vi "MAIN - Quick VIew.vi"() -> ()   [LabVIEW 2014, in "QuickVIew.lvlib"]
uses:
  QuickVIew.lvlib
  Components/System Triggers.ctl
  Components/State Declaration.ctl
  Components/Tree Control/Typedef/TYPEDEF - DataStore Command.ctl
  <vilib>/Utility/error.llb/DialogTypeEnum.ctl
  <vilib>/NI/AMC/Read Termination Message.vi
  <vilib>/NI/AMC/Update Message Routing Info.vi
  <vilib>/NI/AMC/Create Multiple Messages.vi
  <vilib>/NI/AMC/Create Single Message.vi
  Components/TypeDef - SHIFTER.ctl
  <vilib>/NI/AMC/Globals.vi
  Components/VI Collection/set Active VIs.vi
  <vilib>/NI/AMC/Send Message.vi
  <vilib>/LabVIEW Icon API/lv_icon/Classes/Icon/Icon.lvclass
  Components/VI Collection/VI Collection.lvclass
  Components/Dependencies.llb/TLB`_Dependencies.lvlib
  <vilib>/NI/AMC/AMC.lvlib
  <vilib>/LabVIEW Icon API/LabVIEW Icon API.lvlib
panel:
  out "Active Icon":picture
  in  "Settings Button":bool
  in  "Unload Button":bool
  in  "Load Button":bool
  in  "Collection View":string(tree)
  in  "DEBUG::VIew Item":enum16{"Block Diagram", "Front Panel", "Icon"}(ring)
  in  "Send Trigger":bool
  in  "System Triggers":T1=enum."Load Selection"
  out "error out":errorcluster
  # "Quick VIew"
  # "Debug Pane"
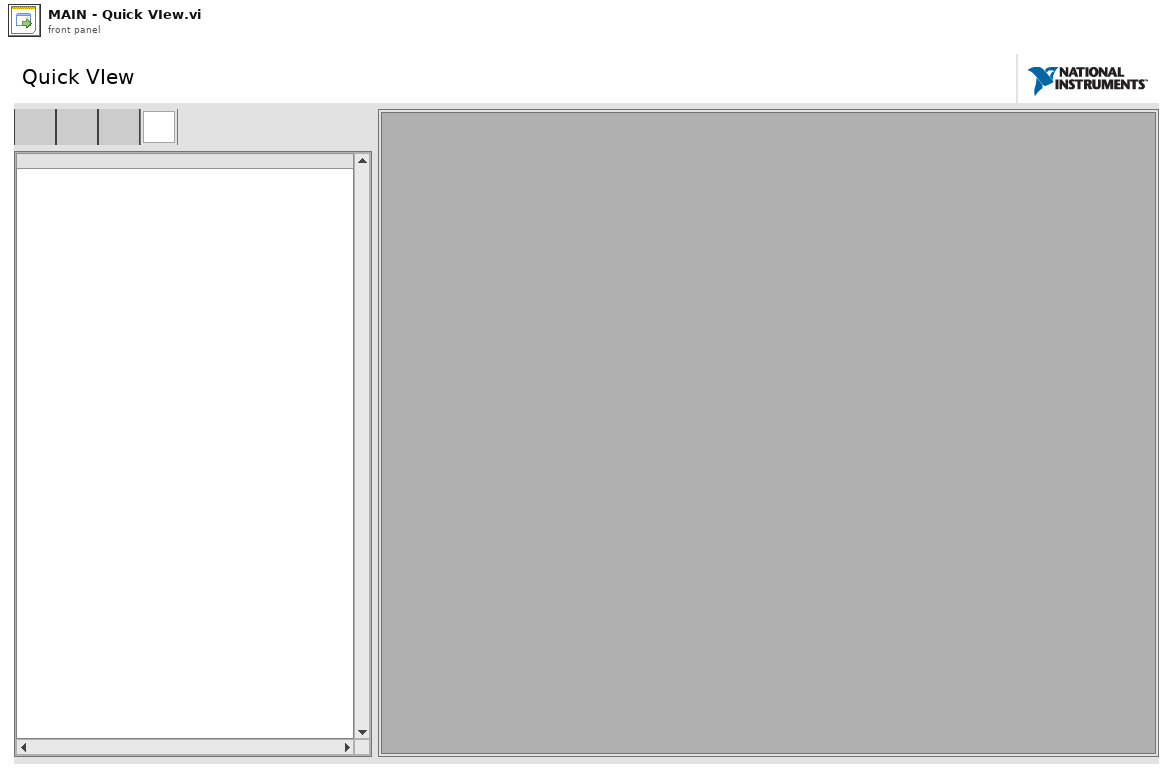
[diagram p1: front panel]
types:
  T1 = typedef "QuickVIew.lvlib/System Triggers.ctl" = enum16{"<None>", "Cache User Parameters", "Close Application", "---------------------------", "Change VI", "Open Current VI", "Save VI", "Unload Collection", "Load Selection", "Edit Icon"}
  T2 = enum16{"Clear SR", "Set Display", "Set Shifter", "Initialize Events", "Init Q"}
  T3 = typedef "QuickVIew.lvlib/TypeDef - SHIFTER.ctl" = cluster{"State":T4, "User Data":cluster{"Active Item Tag":string}, "Display Data":cluster{"Current Project Name":string, "Active Icon":picture}, "User Parameter Controls":refnum<vi>[], "Framework Data":cluster{"Exit Event":T5, "Terminate Error":errorcluster}, "Private Data":cluster{"Active Item Tag":string, "Scroll Event":refnum<user-event>, "ActiveProject":refnum<vi>, "Active VI":cluster{"App Ref":refnum<vi>, "VI Name":string, "Active Window":enum16{"FP", "BD"}, "Icon":refnum<class "Icon.lvclass">}, "Loaded VI":refnum<vi>, "Collection View Tree":refnum<vi>, "Item View":refnum<vi>, "VI Collection":refnum<class "VI Collection.lvclass">}}
  T4 = typedef "QuickVIew.lvlib/State Declaration.ctl" = enum16{"<Startup>", "Idle", "<Shutdown>", "-", "Viewing"}
  T5 = typedef "QuickVIew.lvlib/TLB`_Dependencies.lvlib/Exit Event Ref.ctl" = refnum<user-event>
  T6 = typedef "AMC.lvlib/Message Queue.ctl" = refnum<queue>
  T7 = typedef "QuickVIew.lvlib/TYPEDEF - DataStore Command.ctl" = enum16{"Init", "Add", "Get", "Clear Tree", "Clear All", "Modify"}
  T8 = enum32{"Invalid", "Standard", "Closed", "Hidden", "Minimized", "Maximized"}
  T9 = typedef "DialogTypeEnum.ctl" = enum16{"no dialog", "OK message", "continue or stop message", "auto error handling dialog", "OK message + warnings", "continue/stop + warnings"}
  T10 = typedef "imagedata.ctl" = cluster{"image type":i32, "image depth":i32, "image":u8[], "mask":u8[], "colors":u32[], "Rectangle":cluster{"left":i16, "top":i16, "right":i16, "bottom":i16}}
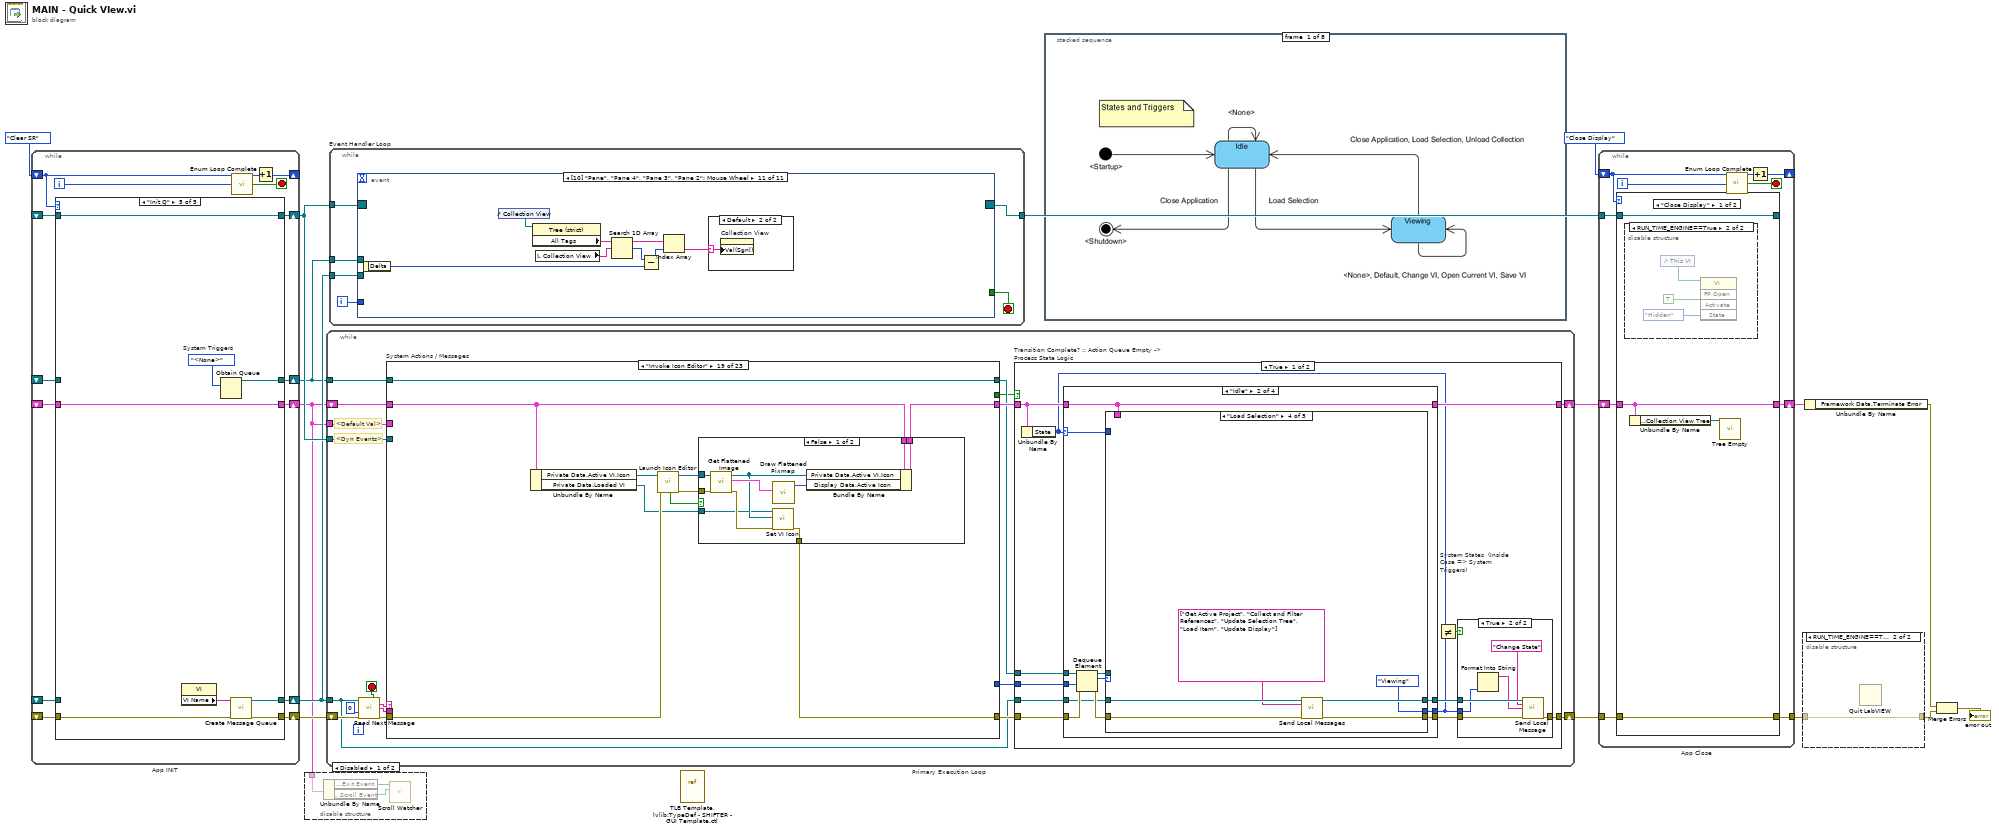
[diagram p0: block diagram]
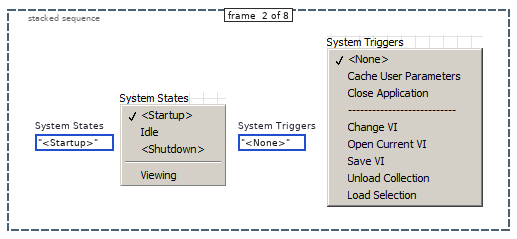
[diagram p3: hidden frame]
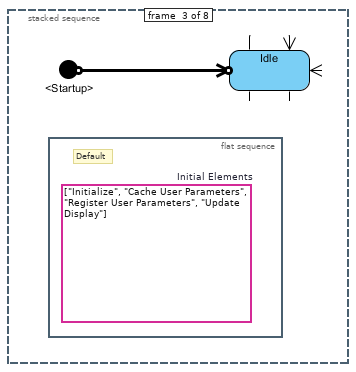
[diagram p4: hidden frame]
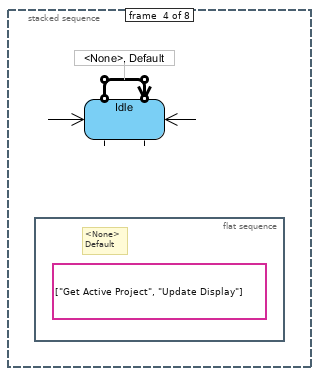
[diagram p5: hidden frame]
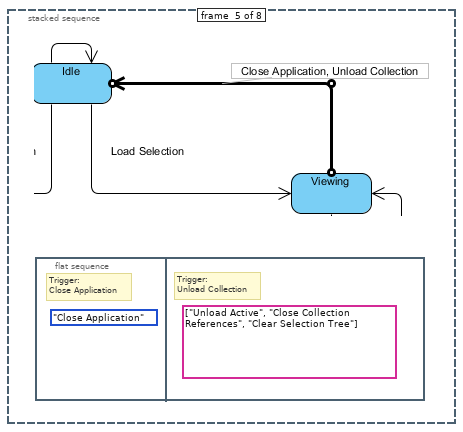
[diagram p6: hidden frame]
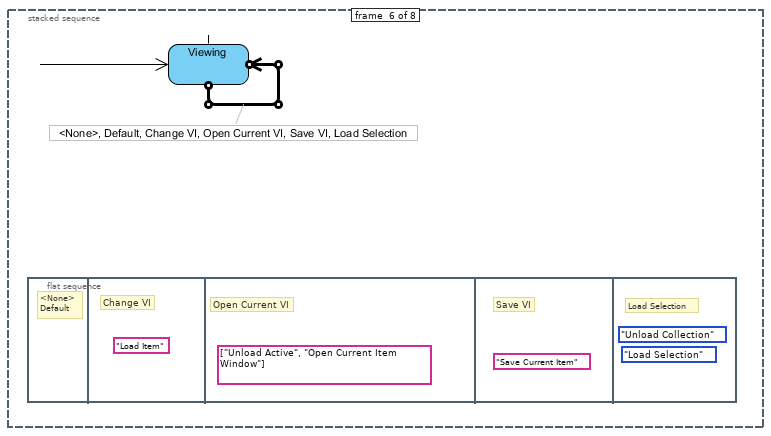
[diagram p7: hidden frame]
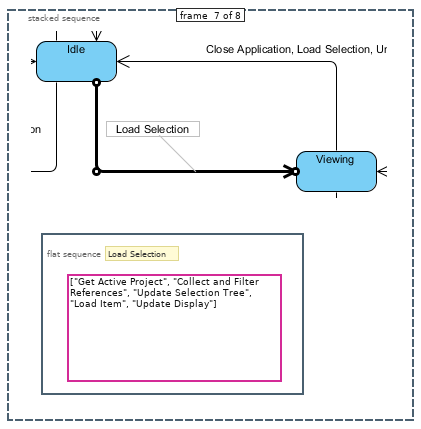
[diagram p8: hidden frame]
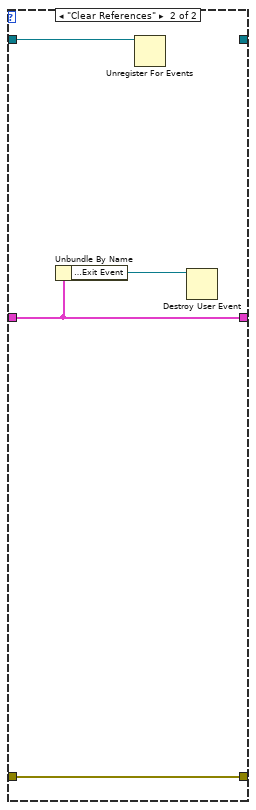
[diagram p12: hidden frame]
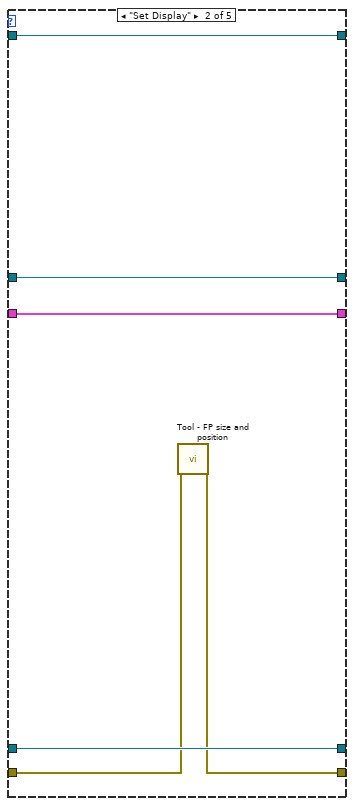
[diagram p14: hidden frame]
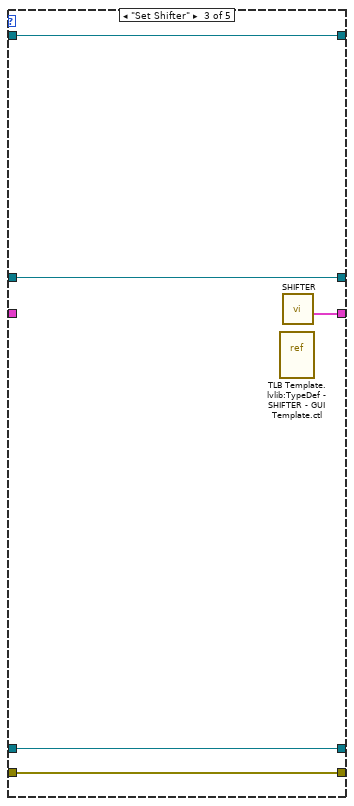
[diagram p15: hidden frame]
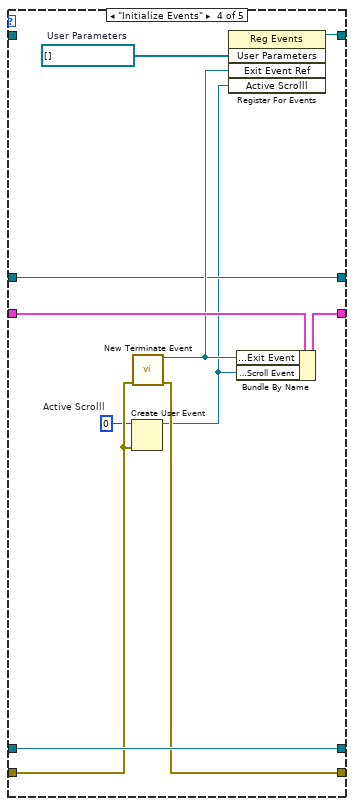
[diagram p16: hidden frame]
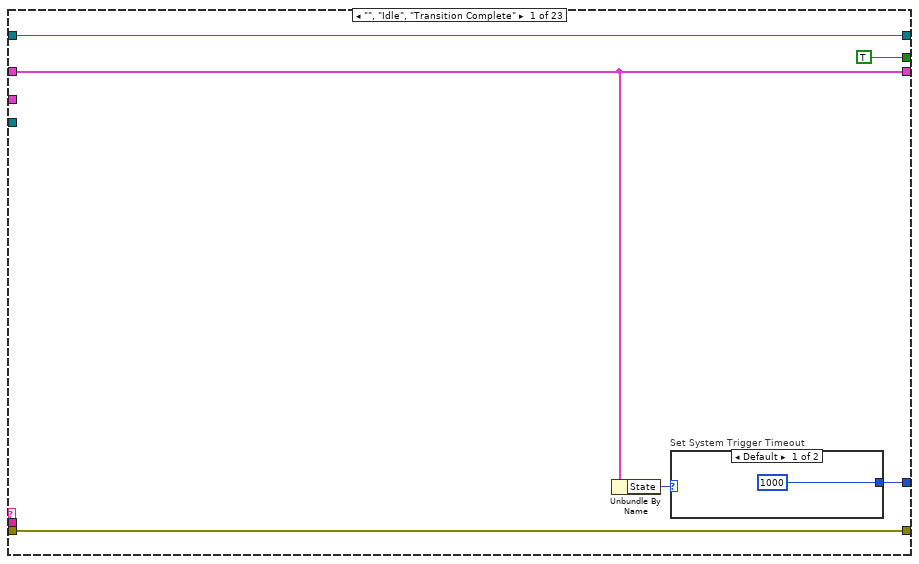
[diagram p17: hidden frame]
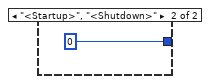
[diagram p18: hidden frame]
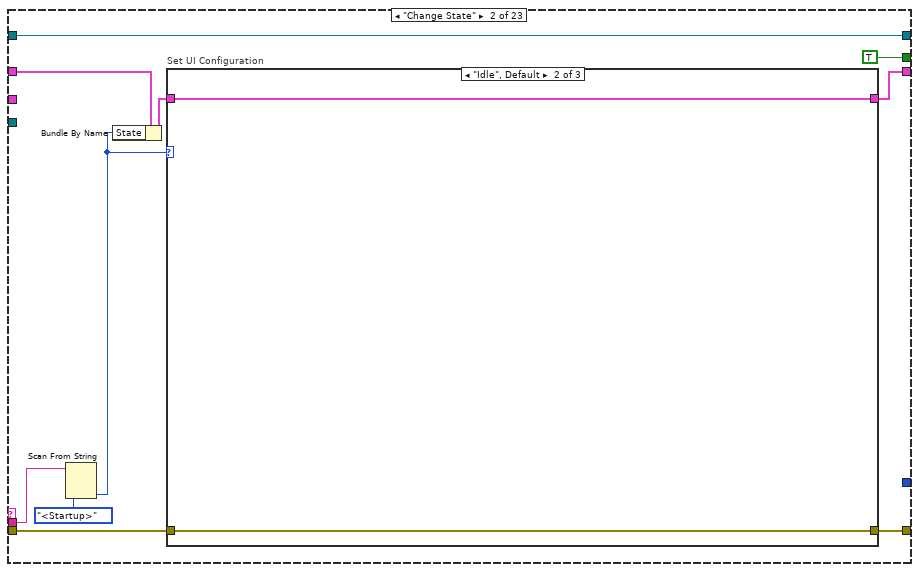
[diagram p19: hidden frame]
diagram:
  n1 = while "App INIT" {
    shift-right: [w23] -> _
    shift-left: T2."Clear SR" -> [w18]
    shift-right: [w29] -> w9
    shift-left: _ -> [w22]
    shift-right: [w26] -> w8
    shift-left: _ -> [w21]
    shift-right: [w28] -> w11
    shift-left: _ -> [w20]
    shift-right: [w27] -> w1
    shift-left: _ -> [w19]
    shift-right: [w17] -> w2
    shift-left: _ -> [w16]
    i -> [w24]
    stop <- w25 stop-if-true
    n2 = case shown="\"Init Q\"" w18 {
      tunnel: [_ w33 w40 w51 w56] -> w29
      tunnel: [_ w31 w39 w45 w54] -> w26
      tunnel: [_ w35 w36 w48 w58] -> w27
      tunnel: [_ w34 w38 w47 w59] -> w28
      tunnel: w22 -> [_ w33 w40 w51 _]
      tunnel: w21 -> [_ w32 w39 w43 w55]
      tunnel: w20 -> [_ w34 w38 _ w59]
      tunnel: w19 -> [_ w35 _ w49 w58]
      tunnel: [_ w30 w37 w44 w53] -> w17
      tunnel: w16 -> [_ w30 w37 w44 _]
      frame "Clear SR" {
      }
      frame "Set Display" {
        n3 = call "Tool - FP size and position.vi"("error in (no error)"=w32) -> ("error out"=w31:errorcluster)  [unwired: 7 in, 11 out]
      }
      frame "Set Shifter" {
        n4 = vi-ref "TLB Template.lvlib:TypeDef - SHIFTER - GUI Template.ctl"() -> ()  [unwired: 1 out]
        n5 = call "SHIFTER.vi"() -> ("SHIFTER DATA"=w36:T3)  [unwired: 15 in]
      }
      frame "Initialize Events" {
        w41 = i16 0  # Active Scrolll
        w50 = refnum<vi>[] []  # User Parameters
        n6 = Create User Event(user event datatype=w41, error in=w43) -> (user event=w42:refnum<user-event>)  [unwired: 1 out]
        n7 = call "New Terminate Event.vi"("error in (no error)"=w43) -> ("Exit Event Ref"=w46:T5, "error out"=w45:errorcluster)  [unwired: 13 in]
        n8 = register-events(w50, w46, w42) -> (reference out=w47:refnum<event-registration>)  [unwired: 2 in, 1 out]
        n9 = Bundle By Name(cluster=w49, "Framework Data.Exit Event"=w46, "Private Data.Scroll Event"=w42) -> (w48:T3)
      }
      frame "Init Q" {
        w52 = System_Triggers."<None>"  # System Triggers
        n10 = property class="VI"() -> ("VI Name"=w57:string)  [unwired: 2 in, 2 out]
        n11 = Obtain Queue(element data type=w52) -> (queue out=w53:refnum<queue>)  [unwired: 4 in, 2 out]
        n12 = call <vilib>:"Create Message Queue.vi"("message queue name"=w57, "error in"=w55) -> ("message queue out"=w56:T6, "error out"=w54:errorcluster)  [unwired: 12 in]
      }
    }
    n13 = call "Enum Loop Complete.vi"("Current State Enum"=w18, "Itteration"=w24) -> ("Loop Complete?"=w25:bool)  [unwired: 13 out]
    n14 = Increment(x=w18) -> (x+1=w23:T2)
  }
  n15 = disable-structure shown="Disabled" {
    disable-tunnel: w1 -> [w62 _]
    frame Disabled {
      n16 = Unbundle By Name(w62) -> ("Framework Data.Exit Event"=w61:T5, "Private Data.Scroll Event"=w60:refnum<user-event>)
      n17 = call "Scroll Watcher.vi"("Exit Command"=w61, "NewVal"=w60) -> ()  [unwired: 14 in]
    }
    frame Enabled {
    }
  }
  n18 = while "Primary Execution Loop" {
    shift-right: [w70] -> w15
    shift-left: w8 -> [w77]
    shift-right: [w73] -> w14
    shift-left: w1 -> [w80]
    tunnel: w1 -> [w79]
    tunnel: w9 -> [w68]
    tunnel: w11 -> [w78]
    tunnel: w2 -> [w69]
    stop <- w75 stop-if-true
    # "<Dyn Events>"
    # "<Default Val>"
    n19 = call <vilib>:"Read Next Message.vi"("message queue in"=w68, "timeout (1 ms)"=0 ("timeout (1ms)"), "error in"=w77) -> ("exit process?"=w75:bool, "message name"=w74:string, "message value"=w65:string, "error out"=w76:errorcluster)  [unwired: 5 in, 4 out]
    n20 = case "System Actions / Messages" shown="\"Invoke Icon Editor\"" w74 {
      selector: w74 -> [_ _ _ _ _ _ _ _ _ _ _ _ _ _ _ _ _ _ _ _ _ _ w345]
      tunnel: [w86 w93 w107 w113 w122 w125 w130 w134 w137 w140 w189 w200 w219 w249 w261 w278 w281 w282 w290 w311 w316 w339 w349] -> w71
      tunnel: w76 -> [w86 w92 w107 w114 w122 w125 w130 w134 w137 w141 w190 w201 w220 w250 w262 w278 w281 w283 w295 w311 w317 w338 w350]
      tunnel: w80 -> [w81 w89 w106 w111 w121 w124 w128 w132 w136 w139 w194 w205 w229 w251 w263 w275 w280 w284 w294 w310 w314 w342 w351]
      tunnel: w79 -> [_ _ _ _ _ _ _ _ _ _ _ _ _ _ _ _ _ _ _ _ _ _ _]
      tunnel: [w81 w91 w106 w110 w120 w124 w127 w132 w136 w142 w193 w204 w228 w251 w263 w275 w280 w284 w293 w310 w315 w342 w351] -> w72
      tunnel: [w82 _ _ _ _ _ _ _ _ _ _ _ _ _ _ _ _ _ _ _ _ _ _] -> w64
      tunnel: w78 -> [_ _ _ _ w119 _ _ _ _ _ _ _ _ _ _ _ _ _ _ _ _ _ _]
      tunnel: [w84 w97 w105 w115 w118 w123 w129 w133 w135 w150 w197 w210 w241 w260 w274 w277 w279 w286 w296 w309 w312 w336 w343] -> w67
      tunnel: w69 -> [w84 w97 w105 w115 w118 w123 w129 w133 w135 w150 w197 w210 w241 w260 w274 w277 w279 w286 w296 w309 w312 w336 w343]
      tunnel: [TRUE TRUE _ _ _ _ _ _ _ _ _ _ _ _ _ _ _ _ _ _ _ _ _] -> w66
      tunnel: w65 -> [_ w96 _ _ _ _ _ _ _ _ _ _ _ _ _ _ _ _ _ _ _ _ _]
      frame "", "Idle", "Transition Complete" {
        n21 = Unbundle By Name(w81) -> ("State"=w83:T4)
        n22 = case "Set System Trigger Timeout" shown="Default" w83 {
          tunnel: [1000 0] -> w82
          frame Default {
          }
          frame "<Startup>", "<Shutdown>" {
          }
        }
      }
      frame "Change State" {
        n23 = Scan From String(input string=w96, default 1=State_Declaration."<Startup>" ("State")) -> (output 1=w94:T4)  [unwired: 3 in, 3 out]
        n24 = Bundle By Name(cluster=w89, "State"=w94) -> (w90:T3)
        n25 = case "Set UI Configuration" shown="\"Idle\", Default" w94 {
          tunnel: [w99 w102 w104] -> w93
          tunnel: w92 -> [w99 w102 w104]
          tunnel: [w100 w101 w103] -> w91
          tunnel: w90 -> [w100 w101 w103]
          frame "<Startup>" {
          }
          frame "Idle", Default {
          }
          frame "<Shutdown>" {
          }
        }
      }
      frame "/*********Initialize********/" {
      }
      frame "Initialize" {
        n26 = control-ref of="Collection View"() -> (w112:refnum<vi>)
        n27 = control-ref of="View Panel"() -> (w108:refnum<vi>)
        n28 = call "Tree Empty.vi"("Tree Reference In"=w112, "error in (no error)"=w114) -> ("Tree Reference Out"=w109:refnum<vi>, "error out"=w113:errorcluster)  [unwired: 15 in, 1 out]
        n29 = Bundle By Name(cluster=w111, "Private Data.Item View"=w108, "Private Data.Collection View Tree"=w109) -> (w110:T3)
      }
      frame "Register User Parameters" {
        n30 = control-ref of="Collection View"() -> (w116:refnum<vi>)
        n31 = Build Array(w116) -> (w117:refnum<vi>[])
        n32 = register-events(reference=w119, w117) -> ()  [unwired: 3 in, 2 out]
        n33 = Bundle By Name(cluster=w121, "User Parameter Controls"=w117) -> (w120:T3)
      }
      frame "/*********Display Updates********/" {
      }
      frame "Cache User Parameters" {
        n34 = Bundle By Name(cluster=w128, "User Data.Active Item Tag"="Collection View") -> (w127:T3)
      }
      frame "Update Display" {
        n35 = Unbundle By Name(w132) -> ("Display Data.Active Icon"=→"Active Icon":picture)
      }
      frame "/*********Primary Execution********/" {
      }
      frame "Get Active Project" {
        n36 = Unbundle By Name(w139) -> ("Display Data.Current Project Name"=w149:string, "Private Data.ActiveProject"=w146:refnum<vi>)
        n37 = property class="App"(error in=w141) -> (error out=w143:errorcluster, "Project.ActiveProject"=w144:refnum<vi>)  [unwired: 1 in, 1 out]
        n38 = while {
          tunnel: w139 -> [w152]
          tunnel: [w151] -> w138
          stop <- w153 stop-if-true
          n39 = event shown="[1] VI Activation" {
            selector: _ -> [_ _]
            dyn-events: _ -> [_ _]
            timeout: 0 -> [_ _]
            tunnel: [TRUE TRUE] -> w153
            tunnel: w152 -> [w155 w159]
            tunnel: [w155 w158] -> w151
            event Timeout {
              n40 = event-data() -> ()  [unwired: 1 in, 1 out]
            }
            event VI Activation {
              n41 = event-data() -> ("VIName"=w160:string, "VIAppRef"=w161:refnum<vi>, "VIWindow"=w164:i32)  [unwired: 1 in]
              n42 = property class="VI"() -> ("Name"=w163:string)  [unwired: 2 in, 2 out]
              n43 = Equal?(x=w160, y=w163) -> (x = y?=w162:bool)
              n44 = case shown="False" w162 {
                tunnel: w164 -> [w166 w174]
                tunnel: w161 -> [w167 _]
                tunnel: w160 -> [w168 _]
                tunnel: w159 -> [w170 w173]
                tunnel: [w169 w173] -> w158
                frame False {
                  n45 = case shown="1" w166 {
                    tunnel: [enum16{"FP", "BD"}."FP" enum16{"FP", "BD"}."BD"] -> w165
                    frame 0, Default {
                    }
                    frame 1 {
                    }
                  }
                  n46 = Bundle By Name(cluster=w170, "Private Data.Active VI.VI Name"=w168, "Private Data.Active VI.App Ref"=w167, "Private Data.Active VI.Active Window"=w165) -> (w169:T3)
                }
                frame True {
                  n47 = case shown="1" w174 {
                    tunnel: [enum16{"FP", "BD"}."FP" enum16{"FP", "BD"}."BD"] -> _
                    frame 0, Default {
                    }
                    frame 1 {
                    }
                  }
                }
              }
            }
          }
        }
        n48 = Equal?(x=w146, y=w144) -> (x = y?=w145:bool)
        n49 = case "is active project ref unchanged?" shown="True" w145 {
          tunnel: w144 -> [w182 w188]
          tunnel: w146 -> [w178 w187]
          tunnel: [w180 w187] -> w147
          tunnel: [w181 w186] -> w140
          tunnel: w143 -> [w183 w185]
          tunnel: [w179 w184] -> w148
          tunnel: w149 -> [_ w184]
          frame False {
            n50 = property class="Project"(reference=w182, error in=w183) -> (reference out=w180:refnum<vi>, error out=w181:errorcluster, "Name"=w179:string)
            n51 = Close Reference(reference=w178, error in (no error)=w183) -> (error out=w177:errorcluster)
            n52 = call <vilib>:"Clear Errors.vi"("error in (no error)"=w177) -> ()  [unwired: 5 in, 2 out]
          }
          frame True {
            n53 = Close Reference(reference=w188, error in (no error)=w185) -> (error out=w186:errorcluster)
          }
        }
        n54 = Bundle By Name(cluster=w138, "Display Data.Current Project Name"=w148, "Private Data.ActiveProject"=w147) -> (w142:T3)
      }
      frame "Collect and Filter References" {
        n55 = Unbundle By Name(w194) -> ("Private Data.VI Collection"=w196:refnum<class "VI Collection.lvclass">, "Private Data.ActiveProject"=w192:refnum<vi>)
        n56 = call "Harvest Selected Project Vi.vi"("ActiveProject"=w192, "error in"=w190) -> ("Array"=w191:refnum<vi>[], "error out"=w198:errorcluster)  [unwired: 12 in]
        n57 = property class="VI Collection"(reference=w196, error in=w198, "Active VIs"=w191) -> (reference out=w195:refnum<class "VI Collection.lvclass">, error out=w189:errorcluster)
        n58 = Bundle By Name(cluster=w194, "Private Data.VI Collection"=w195) -> (w193:T3)
      }
      frame "Update Selection Tree" {
        n59 = Unbundle By Name(w205) -> ("Private Data.Collection View Tree"=w206:refnum<vi>, "Private Data.VI Collection"=w199:refnum<class "VI Collection.lvclass">)
        n60 = call "get Names.vi"("error in (no error)"=w201, "VI Collection in"=w199) -> ("error out"=w202:errorcluster, "VI Ref"=w208:refnum<vi>[], "VI Names"=w207:string[])  [unwired: 6 in, 1 out]
        n61 = for {
          tunnel: w206 -> [w216]
          tunnel: w207 -> [w215] mode=indexing
          tunnel: w208 -> [w214] mode=indexing
          tunnel: [w213] -> w209 mode=indexing
          shift-right: [w211] -> w200
          shift-left: w202 -> [w212]
          n62 = call "Item Add.vi"("Tree Reference In"=w216, "New Text Value"=w215, "Tree Element Data In"=w214, "error in (no error)"=w212, "Make Top Level Item"=TRUE) -> ("Created Tag"=w213:string, "error out"=w211:errorcluster)  [unwired: 12 in, 1 out]
        }
        n63 = Index Array(array=w209) -> (element=w203:string)  [unwired: 1 in]
        n64 = local write "Collection View"(w203) -> ()
        n65 = Bundle By Name(cluster=w205, "User Data.Active Item Tag"=w203) -> (w204:T3)
      }
      frame "Load Item" {
        n66 = Unbundle By Name(w229) -> ("Private Data.Collection View Tree"=w232:refnum<vi>, "User Data.Active Item Tag"=w233:string)
        n67 = Unbundle By Name(w229) -> ("Private Data.Item View"=w231:refnum<vi>)
        n68 = call "VIG - Element DB.vi"("Tree Ref In"=w232, "Element Tag"=w233, "error in (no error)"=w220, "Command"=TYPEDEF_-_DataStore_Command."Get") -> ("Tree Element Data Out"=w234:variant, "error out"=w236:errorcluster)  [unwired: 6 in, 4 out]
        n69 = Variant To Data(error in=w236, type=refnum<vi> refnum ("Reference"), Variant=w234) -> (data=w239:refnum<vi>, error out=w240:errorcluster)
        n70 = property class="VI"(reference=w239, error in=w240, "Edit Mode"=TRUE ("Edit Mode On Open")) -> (reference out=w226:refnum<vi>, error out=w223:errorcluster)
        n71 = case shown="\"Block Diagram\", Default" "DEBUG::VIew Item" {
          tunnel: w231 -> [w245 w248]
          tunnel: w223 -> [w244 _]
          tunnel: w226 -> [w242 w247]
          tunnel: [w242 w247] -> w227
          frame "Block Diagram", Default {
            w246 = TRUE ("ShowHScrollBar")
            n72 = invoke on="Invoke Node" class="SubPanel" method="InsertBD"(reference=w245, error in=w244, "VIRef"=w242, "ShowHScrollBar?"=w246, "ShowVScrollBar?"=w246) -> (error out=w243:errorcluster)  [unwired: 1 in, 5 out]
            n73 = call <vilib>:"Clear Errors.vi"("error in (no error)"=w243) -> ()  [unwired: 5 in, 2 out]
          }
          frame "Front Panel" {
            n74 = invoke on="Invoke Node" class="SubPanel" method="Insert VI"(reference=w248, "VI Ref"=w247) -> ()  [unwired: 2 in, 4 out]
          }
        }
        n75 = call <vilib>:"Get VI Icon.vi"("error in (no error)"=w223, "VI Refnum in"=w226) -> ("error out"=w222:errorcluster, "Icon"=w225:refnum<class "Icon.lvclass">)  [unwired: 7 in, 1 out]
        n76 = call <vilib>:"Get Flattened Image.vi"("error in (no error)"=w222, "lv_icon.lvlib:Icon.lvclass in"=w225) -> ("error out"=w219:errorcluster, "Color Image"=w224:T10, "lv_icon.lvlib:Icon.lvclass out"=w218:refnum<class "Icon.lvclass">)  [unwired: 6 in, 1 out]
        n77 = call <vilib>:"Draw Flattened Pixmap.vi"("image data"=w224) -> ("new picture"=w221:picture)  [unwired: 8 in]
        n78 = Bundle By Name(cluster=w229, "Private Data.Loaded VI"=w227, "Private Data.Active VI.Icon"=w218, "Display Data.Active Icon"=w221) -> (w228:T3)
      }
      frame "Save Current Item" {
        n79 = Unbundle By Name(w251) -> ("Private Data.Collection View Tree"=w252:refnum<vi>, "User Data.Active Item Tag"=w253:string)
        n80 = call "VIG - Element DB.vi"("Tree Ref In"=w252, "Element Tag"=w253, "error in (no error)"=w250, "Command"=TYPEDEF_-_DataStore_Command."Get") -> ("Tree Element Data Out"=w254:variant, "error out"=w256:errorcluster)  [unwired: 6 in, 4 out]
        n81 = Variant To Data(error in=w256, type=refnum<vi> refnum ("Reference"), Variant=w254) -> (data=w258:refnum<vi>, error out=w259:errorcluster)
        n82 = invoke on="Invoke Node" class="VI" method="Save.Instrument"(reference=w258, error in=w259) -> (error out=w249:errorcluster)  [unwired: 4 in, 5 out]
      }
      frame "Open Current Item Window" {
        n83 = Unbundle By Name(w263) -> ("Private Data.Collection View Tree"=w264:refnum<vi>, "User Data.Active Item Tag"=w265:string)
        n84 = call "VIG - Element DB.vi"("Tree Ref In"=w264, "Element Tag"=w265, "error in (no error)"=w262, "Command"=TYPEDEF_-_DataStore_Command."Get") -> ("Tree Element Data Out"=w266:variant, "error out"=w268:errorcluster)  [unwired: 6 in, 4 out]
        n85 = Variant To Data(error in=w268, type=refnum<vi> refnum ("Reference"), Variant=w266) -> (data=w270:refnum<vi>, error out=w273:errorcluster)
        n86 = invoke on="Invoke Node" class="VI" method="FP.Open"(reference=w270, error in=w273, "Activate"=TRUE ("Activate?"), "State"=T8."Standard") -> (error out=w261:errorcluster)  [unwired: 1 in, 4 out]
      }
      frame "Unload Active" {
        n87 = Unbundle By Name(w275) -> ("Private Data.Item View"=w276:refnum<vi>)
        n88 = invoke on="Invoke Node" class="SubPanel" method="Remove VI"(reference=w276) -> ()  [unwired: 2 in, 3 out]
      }
      frame "Close Collection References" {
      }
      frame "Clear Selection Tree" {
        n89 = Unbundle By Name(w284) -> ("Private Data.Collection View Tree"=w285:refnum<vi>)
        n90 = call "Tree Empty.vi"("Tree Reference In"=w285, "error in (no error)"=w283) -> ("error out"=w282:errorcluster)  [unwired: 15 in, 2 out]
      }
      frame "Invoke Icon Editor" {
        n91 = Unbundle By Name(w294) -> ("Private Data.Active VI.Icon"=w287:refnum<class "Icon.lvclass">, "Private Data.Loaded VI"=w288:refnum<vi>)
        n92 = call <vilib>:"Launch Icon Editor.vi"("error in (no error)"=w295, "Icon in"=w287) -> ("error out"=w291:errorcluster, "Icon out"=w292:refnum<class "Icon.lvclass">, "Canceled?"=w289:bool)  [unwired: 7 in]
        n93 = case shown="False" w289 {
          tunnel: w294 -> [w306 w307]
          tunnel: [w305 w307] -> w293
          tunnel: w292 -> [w304 _]
          tunnel: w291 -> [w301 w308]
          tunnel: [w298 w308] -> w290
          tunnel: w288 -> [w297 _]
          frame False {
            n94 = call <vilib>:"Get Flattened Image.vi"("error in (no error)"=w301, "lv_icon.lvlib:Icon.lvclass in"=w304) -> ("error out"=w299:errorcluster, "Color Image"=w303:T10, "lv_icon.lvlib:Icon.lvclass out"=w300:refnum<class "Icon.lvclass">)  [unwired: 6 in, 1 out]
            n95 = call <vilib>:"Set VI Icon.vi"("error in (no error)"=w299, "Icon"=w300, "VI Refnum in"=w297) -> ("error out"=w298:errorcluster)  [unwired: 7 in, 1 out]
            n96 = call <vilib>:"Draw Flattened Pixmap.vi"("image data"=w303) -> ("new picture"=w302:picture)  [unwired: 8 in]
            n97 = Bundle By Name(cluster=w306, "Private Data.Active VI.Icon"=w300, "Display Data.Active Icon"=w302) -> (w305:T3)
          }
          frame True {
          }
        }
      }
      frame "/*********Shutdown********/" {
      }
      frame "Error" {
        n98 = Unbundle By Name(w314) -> ("State"=w313:T4)
        n99 = case shown="Default" w313 {
          tunnel: w317 -> [w325]
          tunnel: [w324] -> w316
          tunnel: w314 -> [w321]
          tunnel: [w320] -> w315
          tunnel: w312 -> [w318]
          frame Default {
            n100 = call <vilib>:"General Error Handler CORE.vi"("type of dialog (OK msg:1)"=DialogTypeEnum."auto error handling dialog", "error in (no error)"=w325) -> ("stop event propagated"=w323:bool, "error out"=w319:errorcluster)  [unwired: 12 out]
            n101 = case "User Chose to Stop and Not Continue\nFALSE = Continue: CLEAR ERRORS" shown="True" w323 {
              tunnel: [w326 w330] -> w324
              tunnel: w319 -> [w327 w333]
              tunnel: w321 -> [w328 w335]
              tunnel: [w328 w334] -> w320
              tunnel: w318 -> [_ w331]
              frame False {
                n102 = call <vilib>:"Clear Errors.vi"("error in (no error)"=w327) -> ("error out"=w326:errorcluster)  [unwired: 1 in, 5 out]
              }
              frame True {
                n103 = call <vilib>:"Clear Errors.vi"("error in (no error)"=w333) -> ("error out"=w329:errorcluster)  [unwired: 1 in, 5 out]
                n104 = Bundle By Name(cluster=w335, "Framework Data.Terminate Error"=w333) -> (w334:T3)
                n105 = Enqueue Element(queue=w331, element=System_Triggers."Close Application", error in (no error)=w329) -> (error out=w330:errorcluster)  [unwired: 1 in, 2 out]
              }
            }
          }
        }
      }
      frame "Exit" {
        w337 = refnum<class> refnum  # event data
        # "Don't wire 'Error In'\nMust Execute Regardless"
        n106 = Unbundle By Name(w342) -> ("Framework Data.Exit Event"=w341:T5)  [unwired: 1 out]
        n107 = Generate User Event(user event=w341, event data cluster=w337) -> (error out=w340:errorcluster)  [unwired: 2 in, 1 out]
        n108 = Merge Errors(w340, w338) -> (w339:errorcluster)
      }
      frame Default {
        w347 = 1 items=["No error", "Argument error", "Memory is full", "Out of zone", "End of file", "File already open", "Generic file I/O error", "File not found", "File permission error", "Disk is full", "Duplicate path", "Too many files open", "System feature not enabled", "Resource file not found", "Cannot add resource", "Resource not found", "Image not found", "Image memory error", "Pen does not exist", "Config type invalid", "Config token not found", "Config parse error", "Config memory error", "Bad external code format", "Bad external code offset", "External code not present", "Null window", "Destroy window error", "Null menu", "Print aborted", "Bad print record", "Print driver error", "Windows error during printing", "Memory error during printing", "Print dialog error", "Generic print error", "Invalid device refnum", "Device not found", "Device parameter error", "Device unit error", "Cannot open device", "Device call aborted", "Generic error", "Cancelled by user", "Object ID too low", "Object ID too high", "Object not in heap", "Unknown heap", "Unknown object (invalid DefProc)", "Unknown object (DefProc not in table)", "Message out of range", "Invalid (null) method", "Unknown message", "Manager call not supported", "Bad address", "Network operation in progress", "Network operation timed out", "Connection is busy", "Network attribute not supported", "Network error", "Address in use", "System out of memory", "Connection aborted", "Connection refused", "Not connected", "Already connected", "Connection closed", "Initialization error (interapplication manager)", "Bad occurrence", "Wait on unbound occurrence handler", "Occurrence queue overflow", "Datalog type conflict", "Unused", "Unrecognized type (interapplication manager)", "Memory corrupt", "Failed to make temporary DLL", "Old CIN version", "Drag socket not found", "Failed to load drop-object", "Failed to register OLE object", "Failed to release OLE object", "Format specifier type mismatch", "Unknown format specifier", "Too few format specifiers", "Too many format specifiers", "Scan failed", "Newer CIN version", "Error converting to variant", "Runtime menu error", "Password tampered", "Variant attribute not found", "Incompatible variant data type", "Event data is not available", "Event Store is not present", "Occurrence is not found", "Event Queue is not created", "Event info is not available", "Refnum passed is NULL", "Error retrieving Class GUID", "Error retrieving CoClass GUID", "Error retrieving TypeLib GUID.", "Bad built application magic bytes.", "Specific driver is different from the specific driver associated with the Logical Name.", "There is no session opened to the class driver.", "Max Error", "MAX - Error with config objects", "MAX - Error loading configuration", "MAX - Group not supported"]
        w348 = TRUE  # status
        n109 = Format Into String(format string="DEVELOPER ERROR:\nImproper State Requested\n================\nState {%s} does not exist within this architecture\n\nCheck for spelling and case errors" ("source"), w345) -> (resulting string=w346:string)  [unwired: 2 in, 1 out]
        n110 = Bundle By Name(cluster=w350, "status"=w348, "code"=w347, "source"=w346) -> (w349:errorcluster)
      }
    }
    n111 = case "Transition Complete? :: Action Queue Empty -> Process State Logic" shown="True" w66 {
      tunnel: [w363 w501] -> w73
      tunnel: w72 -> [w353 w501]
      tunnel: w71 -> [w362 w500]
      tunnel: w68 -> [w361 _]
      tunnel: [w357 w500] -> w70
      tunnel: w67 -> [w360 _]
      tunnel: w64 -> [w354 _]
      frame True {
        n112 = Unbundle By Name(w353) -> ("State"=w352:T4)
        n113 = case "System States  (Inside Case => System Triggers)" shown="\"Idle\"" w352 {
          selector: w352 -> [_ w378 w414 _]
          tunnel: [w377 w388 w424 w491] -> w363
          tunnel: w353 -> [w377 w388 w424 w491]
          tunnel: w362 -> [w371 w382 w418 w485]
          tunnel: w361 -> [w373 w380 w416 w483]
          tunnel: [w376 w387 w423 w490] -> w358
          tunnel: w360 -> [_ w389 w425 w493]
          tunnel: [w375 w386 w422 w489] -> w359
          tunnel: [State_Declaration."Idle" ("State") w385 w421 w488] -> w356
          tunnel: w354 -> [_ w383 w419 w487]
          frame "<Startup>" {
            w372 = string[] ["Initialize", "Cache User Parameters", "Register User Parameters", "Update Display"]  # Initial Elements
            n114 = call <vilib>:"Send Local Messages.vi"("message queue in"=w373, "message names"=w372, "error in"=w371) -> ("message queue out"=w375:T6, "error out"=w376:errorcluster)  [unwired: 10 in, 1 out]
          }
          frame "Idle" {
            n115 = Dequeue Element(queue=w389, timeout in ms (-1)=w383, error in (no error)=w382) -> (queue out=w379:refnum<queue>, element=w384:T1, error out=w381:errorcluster)  [unwired: 1 out]
            n116 = case shown="\"Load Selection\"" w384 {
              tunnel: w388 -> [_ _ _ _ _]
              tunnel: [w392 w397 w401 w407 w412] -> w387
              tunnel: w381 -> [w395 w397 w404 w410 w412]
              tunnel: w380 -> [w394 w398 w403 w409 w413]
              tunnel: [w393 w398 w402 w408 w413] -> w386
              tunnel: [w390 State_Declaration."<Shutdown>" ("State") w399 State_Declaration."Viewing" ("State") State_Declaration."Idle" ("State")] -> w385
              tunnel: w379 -> [_ _ _ _ _]
              tunnel: w378 -> [w390 _ w399 _ _]
              frame "<None>" {
                n117 = call <vilib>:"Send Local Messages.vi"("message queue in"=w394, "message names"=string[] ["Get Active Project", "Update Display"], "error in"=w395) -> ("message queue out"=w393:T6, "error out"=w392:errorcluster)  [unwired: 10 in, 1 out]
              }
              frame "Close Application" {
              }
              frame "Cache User Parameters" {
                n118 = call <vilib>:"Send Local Message.vi"("message queue in"=w403, "message name"="Cache User Parameters" ("Message Name"), "error in"=w404) -> ("message queue out"=w402:T6, "error out"=w401:errorcluster)  [unwired: 10 in, 1 out]
              }
              frame "Load Selection" {
                n119 = call <vilib>:"Send Local Messages.vi"("message queue in"=w409, "message names"=string[] ["Get Active Project", "Collect and Filter References", "Update Selection Tree", "Load Item", "Update Display"], "error in"=w410) -> ("message queue out"=w408:T6, "error out"=w407:errorcluster)  [unwired: 10 in, 1 out]
              }
              frame Default {
              }
            }
          }
          frame "Viewing" {
            n120 = Dequeue Element(queue=w425, timeout in ms (-1)=w419, error in (no error)=w418) -> (queue out=w415:refnum<queue>, element=w420:T1, error out=w417:errorcluster)  [unwired: 1 out]
            n121 = case shown="\"Cache User Parameters\"" w420 {
              tunnel: w424 -> [_ _ _ _ _ _ _ _ _ _ _]
              tunnel: [w427 w431 w438 w441 w445 w452 w454 w460 w466 w472 w478] -> w423
              tunnel: w417 -> [w427 w434 w438 w441 w445 w452 w457 w463 w469 w475 w481]
              tunnel: w416 -> [w428 w433 w439 w442 w444 w451 w456 w462 w468 w474 w480]
              tunnel: [w428 w432 w439 w442 w444 w451 w455 w461 w467 w473 w479] -> w422
              tunnel: [w426 w429 State_Declaration."Idle" ("State") State_Declaration."Viewing" ("State") w443 State_Declaration."Viewing" ("State") State_Declaration."Viewing" ("State") State_Declaration."Idle" ("State") State_Declaration."Viewing" ("State") State_Declaration."Viewing" ("State") State_Declaration."Viewing" ("State")] -> w421
              tunnel: w415 -> [_ _ w435 _ _ w449 _ _ _ _ _]
              tunnel: w414 -> [w426 w429 _ _ w443 _ _ _ _ _ _]
              frame "<None>" {
              }
              frame "Cache User Parameters" {
                n122 = call <vilib>:"Send Local Message.vi"("message queue in"=w433, "message name"="Cache User Parameters" ("Message Name"), "error in"=w434) -> ("message queue out"=w432:T6, "error out"=w431:errorcluster)  [unwired: 10 in, 1 out]
              }
              frame "Close Application" {
                n123 = Enqueue Element(queue=w435, element=System_Triggers."Close Application") -> ()  [unwired: 2 in, 3 out]
              }
              frame Default {
              }
              frame "---------------------------" {
              }
              frame "Load Selection" {
                w447 = System_Triggers."Load Selection"  # System Triggers
                w448 = System_Triggers."Unload Collection"  # System Triggers
                n124 = Enqueue Element(queue=w449, element=w448) -> (queue out=w450:refnum<queue>)  [unwired: 2 in, 2 out]
                n125 = Enqueue Element(queue=w450, element=w447) -> ()  [unwired: 2 in, 3 out]
              }
              frame "Change VI" {
                n126 = call <vilib>:"Send Local Messages.vi"("message queue in"=w456, "message names"=string[] ["Load Item", "Update Display"], "error in"=w457) -> ("message queue out"=w455:T6, "error out"=w454:errorcluster)  [unwired: 10 in, 1 out]
              }
              frame "Unload Collection" {
                n127 = call <vilib>:"Send Local Messages.vi"("message queue in"=w462, "message names"=string[] ["Unload Active", "Close Collection References", "Clear Selection Tree"], "error in"=w463) -> ("message queue out"=w461:T6, "error out"=w460:errorcluster)  [unwired: 10 in, 1 out]
              }
              frame "Open Current VI" {
                n128 = call <vilib>:"Send Local Messages.vi"("message queue in"=w468, "message names"=string[] ["Unload Active", "Open Current Item Window"], "error in"=w469) -> ("message queue out"=w467:T6, "error out"=w466:errorcluster)  [unwired: 10 in, 1 out]
              }
              frame "Save VI" {
                n129 = call <vilib>:"Send Local Messages.vi"("message queue in"=w474, "message names"=string[] ["Save Current Item"], "error in"=w475) -> ("message queue out"=w473:T6, "error out"=w472:errorcluster)  [unwired: 10 in, 1 out]
              }
              frame "Edit Icon" {
                n130 = call <vilib>:"Send Local Messages.vi"("message queue in"=w480, "message names"=string[] ["Invoke Icon Editor", "Update Display"], "error in"=w481) -> ("message queue out"=w479:T6, "error out"=w478:errorcluster)  [unwired: 10 in, 1 out]
              }
            }
          }
          frame "<Shutdown>", "-" {
            n131 = Dequeue Element(queue=w493, timeout in ms (-1)=w487, error in (no error)=w485) -> (queue out=w486:refnum<queue>, element=w492:T1, error out=w484:errorcluster)  [unwired: 1 out]
            n132 = case shown="\"<None>\", Default" w492 {
              tunnel: w491 -> [_]
              tunnel: [w494] -> w490
              tunnel: w484 -> [w496]
              tunnel: w483 -> [w497]
              tunnel: [w495] -> w489
              tunnel: [State_Declaration."<Shutdown>" ("State")] -> w488
              tunnel: w486 -> [_]
              frame "<None>", Default {
                n133 = call <vilib>:"Send Local Messages.vi"("message queue in"=w497, "message names"=string[] ["Exit"], "error in"=w496) -> ("message queue out"=w495:T6, "error out"=w494:errorcluster)  [unwired: 10 in, 1 out]
              }
            }
          }
        }
        n134 = Not Equal?(x=w352, y=w356) -> (x != y?=w355:bool)
        n135 = case shown="True" w355 {
          tunnel: w359 -> [_ w370]
          tunnel: w358 -> [w364 w369]
          tunnel: [w364 w368] -> w357
          tunnel: w356 -> [_ w366]
          frame False {
          }
          frame True {
            n136 = Format Into String(w366) -> (resulting string=w365:string)  [unwired: 3 in, 1 out]
            n137 = call <vilib>:"Send Local Message.vi"("message queue in"=w370, "message name"="Change State" ("Message Name"), "message value"=w365, "error in"=w369) -> ("error out"=w368:errorcluster)  [unwired: 9 in, 2 out]
          }
        }
      }
      frame False {
      }
    }
  }
  n138 = while "Event Handler Loop" {
    tunnel: w11 -> [w506]
    tunnel: w9 -> [w505]
    tunnel: [w504] -> w13
    tunnel: w2 -> [w502]
    i -> [w503]
    stop <- w507 stop-if-true
    n139 = event shown="[10] \"Pane\", \"Pane 4\", \"Pane 3\", \"Pane 2\": Mouse Wheel" {
      selector: w506 -> [_ _ _ _ _ _ _ _ _ _ _]
      dyn-events: [_ _ _ _ _ _ _ _ _ _ _] -> w504
      timeout: _ -> [_ _ _ _ _ _ _ _ _ _ _]
      tunnel: [_ _ TRUE ("NewVal") _ _ _ _ _ _ _ _] -> w507
      tunnel: w505 -> [_ _ _ _ _ _ _ _ _ _ _]
      tunnel: w503 -> [_ _ _ _ _ _ _ _ _ _ _]
      tunnel: w502 -> [w509 _ w523 w527 w532 w536 w538 w540 w542 w546 _]
      event Panel Close? {
        w510 = TRUE  # Discard?
        n140 = event-data() -> ()  [unwired: 2 out]
        n141 = Enqueue Element(queue=w509, element=System_Triggers."Close Application") -> ()  [unwired: 2 in, 3 out]
        n142 = event-data("Discard?"=w510) -> ()  [unwired: 1 in, 1 out]
      }
      event Mouse Down {
        n143 = event-data() -> ("Button"=w515:u16, "Mods"=w516:cluster{"Double Click":bool, "Menu Key":bool})  [unwired: 1 out]
        n144 = Unbundle By Name(w516) -> ("Double Click"=w512:bool)
        n145 = Equal?(x=u16 2, y=w515) -> (x = y?=w513:bool)
        n146 = And(x=w513, y=w512) -> (x .and. y?=w511:bool)
        n147 = case "Toggle Menu Visibility :: double RIGHT click on logo" shown="True" w511 {
          frame False {
          }
          frame True {
            n148 = property class="VI"() -> (reference out=w521:refnum<vi>, "TB.Visible"=w519:bool, "Front Panel.ShowMenuBar"=w518:bool)  [unwired: 2 in, 1 out]
            n149 = Not(x=w519) -> (.not. x?=w520:bool)
            n150 = Not(x=w518) -> (.not. x?=w517:bool)
            n151 = property class="VI"(reference=w521, "TB.Visible"=w520, "Front Panel.ShowMenuBar"=w517) -> ()  [unwired: 1 in, 2 out]
          }
        }
      }
      event User Event {
        w522 = System_Triggers."Close Application"  # System Triggers
        n152 = event-data() -> ()  [unwired: 2 out]
        n153 = Enqueue Element(queue=w523, element=w522) -> ()  [unwired: 2 in, 3 out]
      }
      event Value Change {
        n154 = event-data() -> ()  [unwired: 2 out]
        n155 = Enqueue Element(queue=w527, element=System_Triggers."Cache User Parameters") -> (queue out=w526:refnum<queue>)  [unwired: 2 in, 2 out]
        n156 = event "use this event case to register a SPEICIFIC 'User Parameter' for a SPECIFIC action" shown="[1] \"Collection View\": Value Change" {
          selector: _ -> [_ _]
          dyn-events: _ -> [_ _]
          timeout: 0 -> [_ _]
          tunnel: w526 -> [_ w530]
          event Timeout {
            n157 = event-data() -> ()  [unwired: 1 in, 1 out]
          }
          event "Collection View": Value Change {
            n158 = event-data() -> ()  [unwired: 1 in, 1 out]
            n159 = Enqueue Element(queue=w530, element=System_Triggers."Change VI") -> ()  [unwired: 2 in, 3 out]
          }
        }
      }
      event "Collection View": Mouse Down {
        n160 = event-data() -> ("Mods.Double Click"=w531:bool)  [unwired: 1 out]
        n161 = case shown="True" w531 {
          tunnel: w532 -> [_ w533]
          frame False {
          }
          frame True {
            n162 = Enqueue Element(queue=w533, element=System_Triggers."Open Current VI") -> ()  [unwired: 2 in, 3 out]
          }
        }
      }
      event "Load Button": Value Change {
        n163 = event-data() -> ()  [unwired: 2 out]
        n164 = Enqueue Element(queue=w536, element=System_Triggers."Load Selection") -> ()  [unwired: 2 in, 3 out]
      }
      event "Unload Button": Value Change {
        n165 = event-data() -> ()  [unwired: 2 out]
        n166 = Enqueue Element(queue=w538, element=System_Triggers."Unload Collection") -> ()  [unwired: 2 in, 3 out]
      }
      event "Settings Button": Value Change {
        # "Not implemented at this time"
        n167 = event-data() -> ()  [unwired: 2 out]
        n168 = Enqueue Element(queue=w540, element=System_Triggers."<None>") -> ()  [unwired: 2 in, 3 out]
      }
      event "Active Icon": Mouse Up {
        n169 = event-data() -> ("Mods.Double Click"=w541:bool)  [unwired: 1 out]
        n170 = case shown="True" w541 {
          tunnel: w542 -> [_ w544]
          frame False {
          }
          frame True {
            n171 = Enqueue Element(queue=w544, element=System_Triggers."Edit Icon") -> ()  [unwired: 2 in, 3 out]
          }
        }
      }
      event "Send Trigger": Value Change {
        n172 = event-data() -> ()  [unwired: 2 out]
        n173 = Enqueue Element(queue=w546, element="System Triggers") -> ()  [unwired: 2 in, 3 out]
      }
      event Mouse Wheel {
        n174 = event-data() -> ("Delta"=w547:i32)  [unwired: 1 out]
        n175 = control-ref of="Collection View"() -> (w553:refnum<vi>)
        n176 = property class="Tree (strict)"(reference=w553) -> ("All Tags"=w549:string[])  [unwired: 1 in, 2 out]
        n177 = local read "Collection View"() -> (w552:string)
        n178 = Search 1D Array(1D array=w549, element=w552) -> (index of element=w551:i32)  [unwired: 1 in]
        n179 = Subtract(x=w551, y=w547) -> (x-y=w550:i32)
        n180 = Index Array(array=w549, index=w550) -> (element=w548:string)
        n181 = case shown="Default" w548 {
          selector: w548 -> [_ w554]
          frame "" {
          }
          frame Default {
            n182 = property on="Collection View" class="Tree (strict)"("Val(Sgnl)"=w554) -> ()  [unwired: 2 in, 2 out]
          }
        }
      }
    }
  }
  n183 = vi-ref "TLB Template.lvlib:TypeDef - SHIFTER - GUI Template.ctl"() -> ()  [unwired: 1 out]
  n184 = stacked-sequence {
    frame #0 {
    }
    frame #1 {
      (unwired) System_Triggers."<None>"  # System Triggers
      (unwired) State_Declaration."<Startup>"  # System States
    }
    frame #2 {
      n185 = flat-sequence {
        frame #0 {
          (unwired) string[] ["Initialize", "Cache User Parameters", "Register User Parameters", "Update Display"]  # Initial Elements
          # "Default"
        }
      }
    }
    frame #3 {
      n186 = flat-sequence {
        frame #0 {
          (unwired) string[] ["Get Active Project", "Update Display"]
          # "<None>\nDefault"
        }
      }
    }
    frame #4 {
      n187 = flat-sequence {
        frame #0 {
          (unwired) System_Triggers."Close Application" ("element")
          # "Trigger:\nClose Application"
        }
        frame #1 {
          (unwired) string[] ["Unload Active", "Close Collection References", "Clear Selection Tree"]
          # "Trigger:\nUnload Collection"
        }
      }
    }
    frame #5 {
      n188 = flat-sequence {
        frame #0 {
          # "<None>\nDefault"
        }
        frame #1 {
          (unwired) "Load Item" ("Message Name")
          # "Change VI"
        }
        frame #2 {
          (unwired) string[] ["Unload Active", "Open Current Item Window"]
          # "Open Current VI"
        }
        frame #3 {
          (unwired) "Save Current Item" ("Message Name")
          # "Save VI"
        }
        frame #4 {
          (unwired) System_Triggers."Load Selection" ("System Triggers")
          (unwired) System_Triggers."Unload Collection" ("System Triggers")
          # "Load Selection"
        }
      }
    }
    frame #6 {
      n189 = flat-sequence {
        frame #0 {
          (unwired) string[] ["Get Active Project", "Collect and Filter References", "Update Selection Tree", "Load Item", "Update Display"]
          # "Load Selection"
        }
      }
    }
    frame #7 {
      n190 = flat-sequence {
        frame #0 {
          # "Close Applicaiton"
        }
      }
    }
  }
  n191 = while "App Close" {
    shift-right: [w561] -> _
    shift-left: enum16{"Close Display", "Clear References"}."Close Display" -> [w560]
    tunnel: w13 -> [w558]
    tunnel: w15 -> [w559]
    tunnel: [w556] -> w7
    shift-right: [w555] -> w5
    shift-left: w14 -> [w557]
    i -> [w562]
    stop <- w563 stop-if-true
    n192 = case shown="\"Close Display\"" w560 {
      tunnel: [w566 w574] -> w556
      tunnel: [w564 w573] -> w555
      tunnel: [w567 _] -> _
      tunnel: w559 -> [w566 w574]
      tunnel: w558 -> [w567 w571]
      tunnel: w557 -> [w564 w573]
      frame "Close Display" {
        n193 = disable-structure shown="RUN_TIME_ENGINE==True" {
          frame condition #0 (active) {
          }
          frame condition #1 {
            n194 = control-ref of="This VI"() -> (w568:refnum<vi>)
            n195 = invoke class="VI" method="FP.Open"(reference=w568, "Activate"=TRUE ("Activate?"), "State"=T8."Hidden") -> ()  [unwired: 2 in, 5 out]
          }
        }
        n196 = Unbundle By Name(w564) -> ("Private Data.Collection View Tree"=w565:refnum<vi>)
        n197 = call "Tree Empty.vi"("Tree Reference In"=w565) -> ()  [unwired: 16 in, 3 out]
      }
      frame "Clear References" {
        n198 = Unbundle By Name(w573) -> ("Framework Data.Exit Event"=w572:T5)
        n199 = Unregister For Events(event registration refnum=w571) -> ()  [unwired: 1 in, 1 out]
        n200 = Destroy User Event(user event=w572) -> ()  [unwired: 1 in, 1 out]
      }
    }
    n201 = call "Enum Loop Complete.vi"("Current State Enum"=w560, "Itteration"=w562) -> ("Loop Complete?"=w563:bool)  [unwired: 13 out]
    n202 = Increment(x=w560) -> (x+1=w561:enum16{"Close Display", "Clear References"})
  }
  n203 = disable-structure shown="RUN_TIME_ENGINE==True" {
    disable-tunnel: [w575 w576] -> w4
    disable-tunnel: w7 -> [w575 w576]
    frame condition #0 (active) {
    }
    frame condition #1 {
      n204 = Quit LabVIEW() -> ()  [unwired: 1 in]
    }
  }
  n205 = Unbundle By Name(w5) -> ("Framework Data.Terminate Error"=w3:errorcluster)
  n206 = Merge Errors(w3, w4) -> (→"error out":errorcluster)
